vi "Test_3_3vdc loading.vi"(6 "VISA resource name":refnum<visa-resource-name>, 7 "Pass so far?":bool, 8 "error in (no error)":errorcluster, 10 "3.3vdc Load ON (y)":bool=TRUE, 11 "Slot":T1) -> (0 "error out":errorcluster, 2 "3.3vdc AP1":dbl, 3 "ADC reading AP1":string, 4 "VISA resource name out":refnum<visa-resource-name>, 5 "Passed?":bool)   [LabVIEW 2024]
uses:
  AP slots to test.ctl
panel:
  out "3.3vdc AP2":dbl
  out "ADC reading ap2":string
  out "read buffer ap2":string
  out "read buffer ap1":string
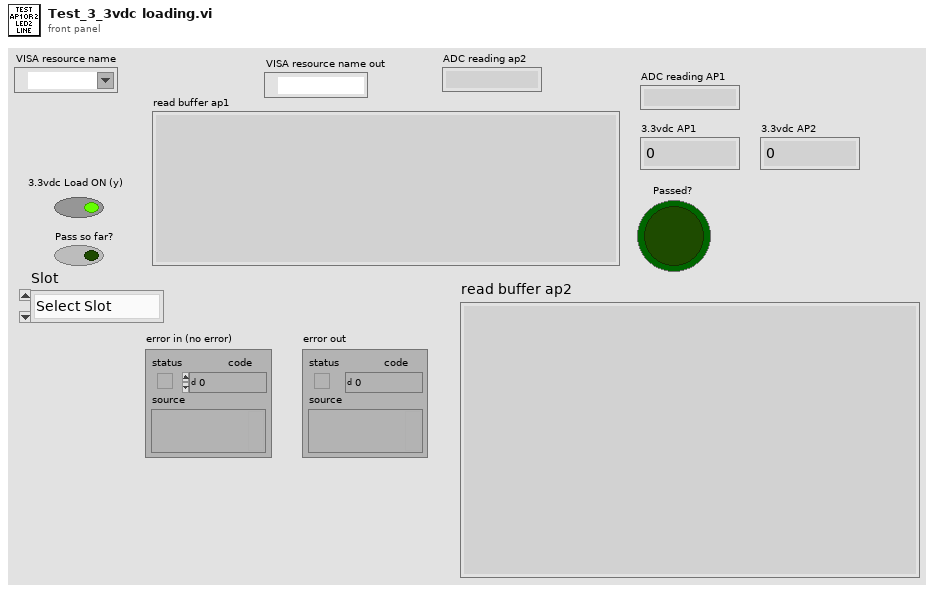
[diagram p1: front panel]
types:
  T1 = typedef "AP slots to test.ctl" = enum16{"Select Slot", "AP1", "AP2", "AP1 and AP2"}
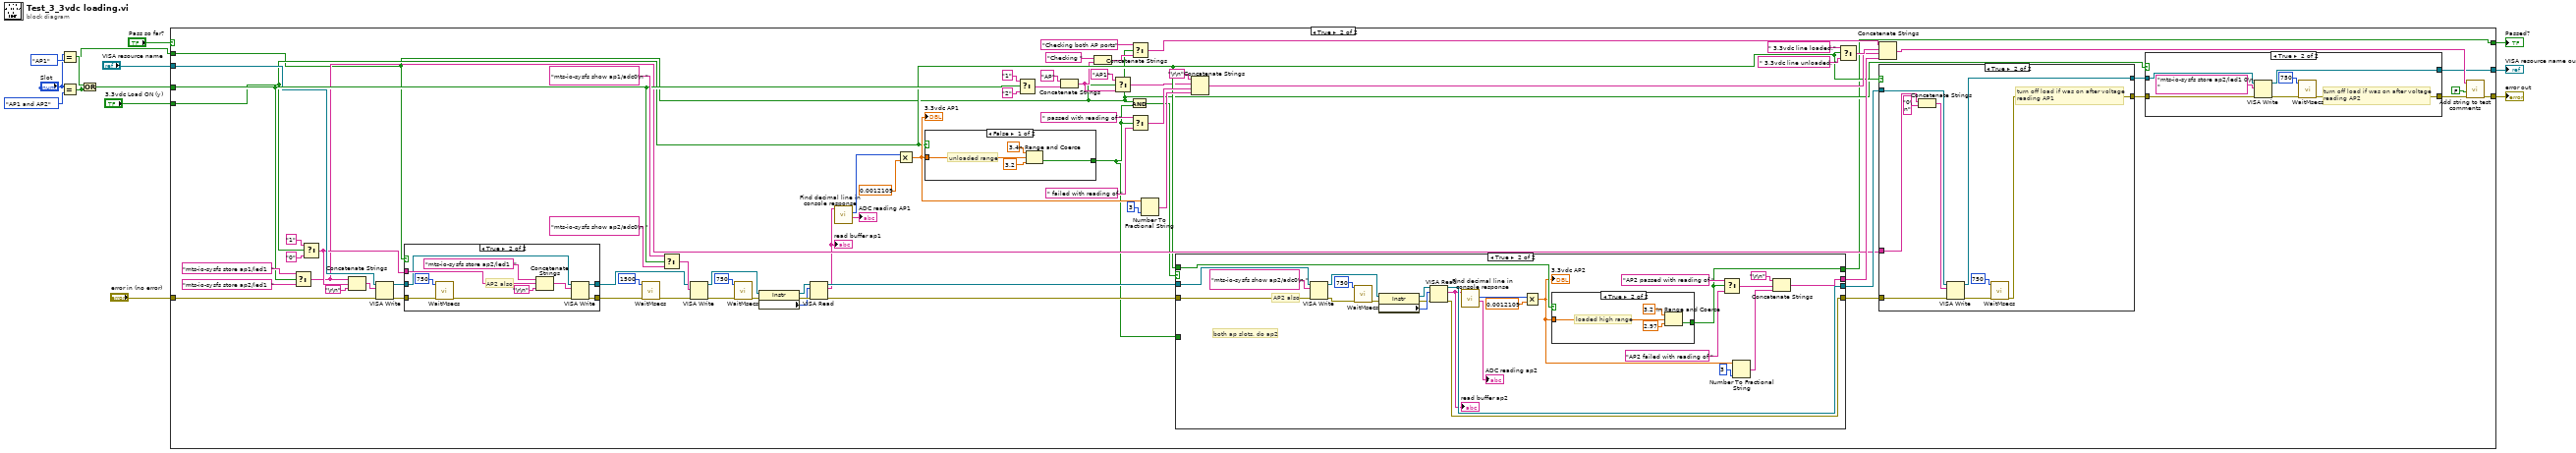
[diagram p0: block diagram]
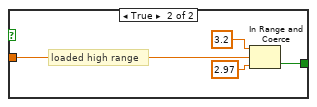
[diagram p3: hidden frame]
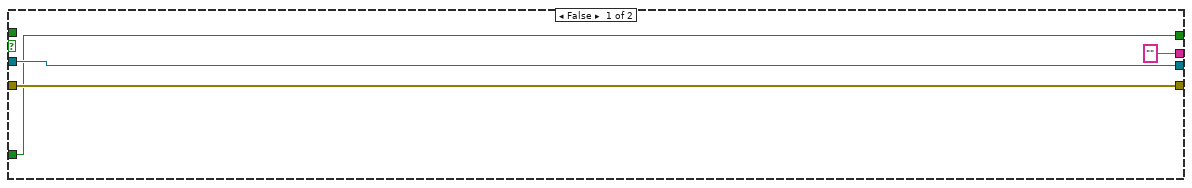
[diagram p5: hidden frame]
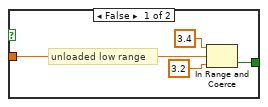
[diagram p6: hidden frame]
diagram:
  n1 = Equal?(x="Slot", y=AP_slots_to_test."AP1") -> (x = y?=w5:bool)
  n2 = Equal?(x="Slot", y=AP_slots_to_test."AP1 and AP2") -> (x = y?=w1:bool)
  n3 = Or(x=w5, y=w1) -> (x .or. y?=w4:bool)
  n4 = case shown="True" "Pass so far?" {
    selector: "Pass so far?" -> [w15 _]
    tunnel: [w16 w58] -> w13
    tunnel: "error in (no error)" -> [w16 w52]
    tunnel: w4 -> [_ w53]
    tunnel: "3.3vdc Load ON (y)" -> [_ w31]
    tunnel: [w15 w18] -> w10
    tunnel: "VISA resource name" -> [w14 w51]
    tunnel: [w14 w38] -> w7
    tunnel: w1 -> [_ w20]
    frame False {
    }
    frame True {
      n5 = Select(t="mts-io-sysfs store ap1/led1  ", s=w53, f="mts-io-sysfs store ap2/led1  ") -> (s? t:f=w32:string)
      n6 = Select(t="1", s=w31, f="0") -> (s? t:f=w50:string)
      n7 = Concatenate Strings(w32, w50, "\r\n") -> (w70:string)
      n8 = VISA Write(VISA resource name=w51, write buffer=w70, error in (no error)=w52) -> (VISA resource name out=w48:refnum<visa-resource-name>, error out=w49:errorcluster)  [unwired: 1 out]
      n9 = case shown="True" w20 {
        tunnel: w50 -> [_ w152]
        tunnel: w49 -> [w143 w145]
        tunnel: w48 -> [w142 w150]
        tunnel: [w143 w148] -> w47
        tunnel: [w142 w147] -> w46
        frame False {
        }
        frame True {
          # "AP2 also"
          n10 = call "WaitMsecs.vi"("error in (no error)"=w145, "Wait Msecs"=u32 750) -> ("error out"=w144:errorcluster)  [unwired: 9 in]
          n11 = Concatenate Strings("mts-io-sysfs store ap2/led1  ", w152, "\r\n") -> (w149:string)
          n12 = VISA Write(VISA resource name=w150, write buffer=w149, error in (no error)=w144) -> (VISA resource name out=w147:refnum<visa-resource-name>, error out=w148:errorcluster)  [unwired: 1 out]
        }
      }
      n13 = call "WaitMsecs.vi"("error in (no error)"=w47, "Wait Msecs"=u32 1500) -> ("error out"=w77:errorcluster)  [unwired: 9 in]
      n14 = Select(t="mts-io-sysfs show ap1/adc0\n ", s=w53, f="mts-io-sysfs show ap2/adc0\n ") -> (s? t:f=w78:string)
      n15 = VISA Write(VISA resource name=w46, write buffer=w78, error in (no error)=w77) -> (VISA resource name out=w76:refnum<visa-resource-name>, error out=w74:errorcluster)  [unwired: 1 out]
      n16 = call "WaitMsecs.vi"("error in (no error)"=w74, "Wait Msecs"=u32 750) -> ("error out"=w73:errorcluster)  [unwired: 9 in]
      n17 = property class="Instr"(reference=w76, error in=w73) -> (reference out=w85:refnum<visa-resource-name>, error out=w84:errorcluster, "Serial Settings:Number of Bytes at Serial Port"=w83:u32)
      n18 = VISA Read(VISA resource name=w85, byte count=w83, error in (no error)=w84) -> (VISA resource name out=w44:refnum<visa-resource-name>, read buffer=w23:string, error out=w45:errorcluster)  [unwired: 1 out]
      "read buffer ap1" <- w23
      n19 = call "Find decimal line in console response.vi"("Console response in"=w23) -> ("output decimal line"=→"ADC reading AP1":string, "Decimal Number"=w22:i32)  [unwired: 7 in, 2 out]
      n20 = Multiply(x=w22, y=0.0012109) -> (x*y=w33:dbl)
      "3.3vdc AP1" <- w33
      n21 = case shown="False" w31 {
        tunnel: w33 -> [w88 w93]
        tunnel: [w87 w92] -> w17
        frame False {
          # "unloaded range"
          n22 = In Range and Coerce(upper limit=3.4, x=w88, lower limit=3.2) -> (In Range?=w87:bool)  [unwired: 1 out]
        }
        frame True {
          # "loaded high range"
          n23 = In Range and Coerce(upper limit=3.2, x=w93, lower limit=2.97) -> (In Range?=w92:bool)  [unwired: 1 out]
        }
      }
      n24 = Select(t="1", s=w53, f="2") -> (s? t:f=w37:string)
      n25 = Concatenate Strings("AP" ("string"), w37) -> (w25:string)
      n26 = Concatenate Strings("Checking " ("Comments"), w25) -> (w26:string)
      n27 = Select(t="AP1", s=w20, f=w25) -> (s? t:f=w24:string)
      n28 = Select(t="Checking both AP ports", s=w20, f=w26) -> (s? t:f=w35:string)
      n29 = And(x=w20, y=w17) -> (x .and. y?=w19:bool)
      n30 = Select(t=" passed with reading of ", s=w17, f=" failed with reading of ") -> (s? t:f=w60:string)
      n31 = Number To Fractional String(number=w33, precision (6)=i16 3) -> (F-format string=w59:string)  [unwired: 2 in]
      n32 = case shown="True" w19 {
        tunnel: w45 -> [w106 w126]
        tunnel: w44 -> [w107 w125]
        tunnel: [w106 w122] -> w43
        tunnel: [w107 w121] -> w42
        tunnel: ["" w114] -> w34
        tunnel: w31 -> [_ w113]
        tunnel: [w104 w108] -> w18
        tunnel: w17 -> [w104 _]
        frame False {
        }
        frame True {
          # "both ap slots, do ap2"
          # "AP2 also"
          n33 = VISA Write(VISA resource name=w125, write buffer="mts-io-sysfs show ap2/adc0\n ", error in (no error)=w126) -> (VISA resource name out=w130:refnum<visa-resource-name>, error out=w132:errorcluster)  [unwired: 1 out]
          n34 = call "WaitMsecs.vi"("error in (no error)"=w132, "Wait Msecs"=u32 750) -> ("error out"=w133:errorcluster)  [unwired: 9 in]
          n35 = property class="Instr"(reference=w130, error in=w133) -> (reference out=w127:refnum<visa-resource-name>, error out=w128:errorcluster, "Serial Settings:Number of Bytes at Serial Port"=w129:u32)
          n36 = VISA Read(VISA resource name=w127, byte count=w129, error in (no error)=w128) -> (VISA resource name out=w121:refnum<visa-resource-name>, read buffer=w111:string, error out=w122:errorcluster)  [unwired: 1 out]
          "read buffer ap2" <- w111
          n37 = call "Find decimal line in console response.vi"("Console response in"=w111) -> ("output decimal line"=→"ADC reading ap2":string, "Decimal Number"=w109:i32)  [unwired: 7 in, 2 out]
          n38 = Multiply(x=w109, y=0.0012109) -> (x*y=w112:dbl)
          "3.3vdc AP2" <- w112
          n39 = case shown="True" w113 {
            tunnel: w112 -> [w136 w140]
            tunnel: [w134 w139] -> w108
            frame False {
              # "unloaded low range"
              n40 = In Range and Coerce(upper limit=3.4, x=w136, lower limit=3.2) -> (In Range?=w134:bool)  [unwired: 1 out]
            }
            frame True {
              # "loaded high range"
              n41 = In Range and Coerce(upper limit=3.2, x=w140, lower limit=2.97) -> (In Range?=w139:bool)  [unwired: 1 out]
            }
          }
          n42 = Select(t="AP2 passed with reading of ", s=w108, f="AP2 failed with reading of ") -> (s? t:f=w118:string)
          n43 = Number To Fractional String(number=w112, precision (6)=i16 3) -> (F-format string=w116:string)  [unwired: 2 in]
          n44 = Concatenate Strings("\r\n", w118, w116) -> (w114:string)
        }
      }
      n45 = Concatenate Strings("\r\n", w24, w60, w59) -> (w57:string)
      n46 = Select(t=" 3.3vdc line loaded.", s=w31, f=" 3.3vdc line unloaded. ") -> (s? t:f=w65:string)
      n47 = Concatenate Strings(w35, w65, w57, w34) -> (w56:string)
      n48 = case shown="True" w31 {
        tunnel: w43 -> [w155 w163]
        tunnel: [w155 w160] -> w41
        tunnel: w42 -> [w154 w164]
        tunnel: [w154 w162] -> w40
        tunnel: w32 -> [_ w156]
        frame False {
        }
        frame True {
          # "turn off load if was on after voltage\nreading AP1"
          n49 = Concatenate Strings(w156, "0\n" ("string")) -> (w157:string)
          n50 = VISA Write(VISA resource name=w164, write buffer=w157, error in (no error)=w163) -> (VISA resource name out=w162:refnum<visa-resource-name>, error out=w161:errorcluster)  [unwired: 1 out]
          n51 = call "WaitMsecs.vi"("error in (no error)"=w161, "Wait Msecs"=u32 750) -> ("error out"=w160:errorcluster)  [unwired: 9 in]
        }
      }
      n52 = case shown="True" w20 {
        tunnel: w41 -> [w96 w102]
        tunnel: [w96 w99] -> w39
        tunnel: w40 -> [w95 w103]
        tunnel: [w95 w101] -> w38
        frame False {
        }
        frame True {
          # "turn off load if was on after voltage\nreading AP2"
          n53 = VISA Write(VISA resource name=w103, write buffer="mts-io-sysfs store ap2/led1 0\n  ", error in (no error)=w102) -> (VISA resource name out=w101:refnum<visa-resource-name>, error out=w100:errorcluster)  [unwired: 1 out]
          n54 = call "WaitMsecs.vi"("error in (no error)"=w100, "Wait Msecs"=u32 750) -> ("error out"=w99:errorcluster)  [unwired: 9 in]
        }
      }
      n55 = call "Add string to test comments.vi"("error in (no error)"=w39, "New Section (y)?"=FALSE, "Comments"=w56) -> ("error out"=w58:errorcluster)  [unwired: 7 in, 1 out]
    }
  }
  "error out" <- w13
  "Passed?" <- w10
  "VISA resource name out" <- w7
